vi "AFG Enable Output.vi"(8 "error in (no error)":errorcluster, 10 "Enable Output (T: Enable)":bool=TRUE, 11 "Actor_AFG in":refnum<class "Actor_AFG.lvclass">) -> (0 "error out":errorcluster, 3 "Actor_AFG out":refnum<class "Actor_AFG.lvclass">)   [LabVIEW 2020, in "Actor_AFG.lvlib" / "Actor_AFG.lvclass"]
uses:
  Actor_AFG.lvclass
  C:/Program Files/National Instruments/LabVIEW 2020/vi.lib/ActorFramework/Actor/Actor.lvclass
  AFG_Event.ctl
  Actor_AFG.lvclass/Actor_AFG.ctl
  <vilib>/ActorFramework/Actor/Actor.lvclass/Actor.ctl
  <instrlib>/Tektronix AFG 3000 Series/Tektronix AFG 3000 Series.lvlib
  <vilib>/ActorFramework/Actor/Actor.lvclass
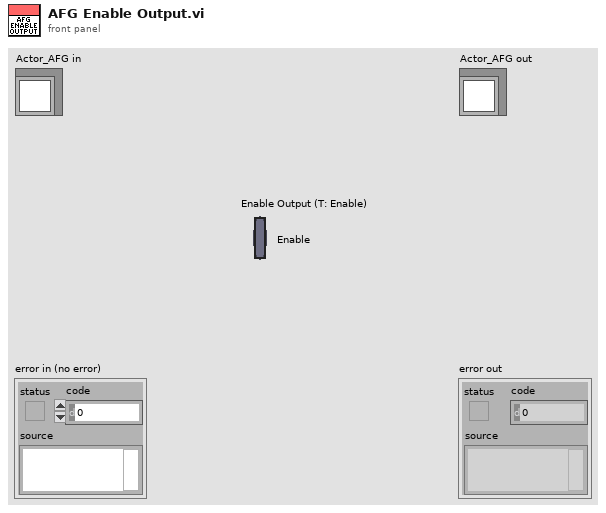
[diagram p1: front panel]
types:
  T1 = typedef "Actor_AFG.lvlib/Actor_AFG.lvclass/AFG_Event.ctl" = enum16{"General Event", "Inited", "Output", "Waveform Set", "Error"}
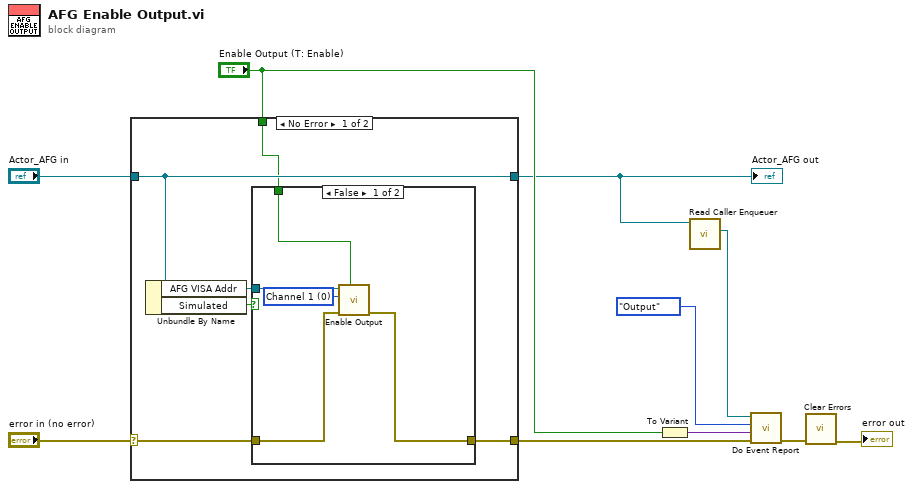
[diagram p0: block diagram]
diagram:
  n1 = case shown="No Error" "error in (no error)" {
    selector: "error in (no error)" -> [w15 w24]
    tunnel: [w14 w24] -> w6
    tunnel: [w16 w23] -> w7
    tunnel: "Actor_AFG in" -> [w16 w23]
    tunnel: "Enable Output (T: Enable)" -> [w11 _]
    frame No Error {
      n2 = Unbundle By Name(w16) -> ("AFG VISA Addr"=w12:refnum<visa-resource-name>, "Simulated"=w13:bool)
      n3 = case shown="False" w13 {
        tunnel: w15 -> [w20 w22]
        tunnel: [w19 w22] -> w14
        tunnel: w12 -> [w21 _]
        tunnel: w11 -> [w17 _]
        frame False {
          w18 = u16 0 items=["Channel 1", "Channel2"] ("Channel (0: Channel 1)")
          n4 = call <instrlib>:"Enable Output.vi"("Enable Output (T: Enable)"=w17, "error in (no error)"=w20, "Channel (0: Channel 1)"=w18, "VISA resource name"=w21) -> ("error out"=w19:errorcluster)  [unwired: 6 in, 1 out]
        }
        frame True {
        }
      }
    }
    frame Error {
    }
  }
  "Actor_AFG out" <- w7
  n5 = To Variant(anything="Enable Output (T: Enable)") -> (Variant=w5:variant)
  n6 = call <vilib>:"Read Caller Enqueuer.vi"("Actor"=w7) -> ("Caller Enqueuer"=w3:refnum<class "Message Enqueuer.lvclass">)  [unwired: 10 in]
  n7 = call "Do Event Report.vi"("error in (no error)"=w6, "Event Data"=w5, "Report Events"=AFG_Event."Output", "Caller Enqueuer"=w3) -> ("error out"=w2:errorcluster)  [unwired: 6 in, 1 out]
  n8 = call <vilib>:"Clear Errors.vi"("error in (no error)"=w2) -> ("error out"=→"error out":errorcluster)  [unwired: 5 in, 1 out]
